vi "Calculate New Account Balance.vi"(6 "Amount":string, 8 "error in (no error)":errorcluster, 11 "Bank Account in":refnum<class "Bank Account.lvclass">) -> (0 "error out":errorcluster, 3 "Bank Account out":refnum<class "Bank Account.lvclass">, 4 "Sufficient Funds?":bool)   [LabVIEW 2016, in "CLD Exam - ATM.lvlib" / "Bank Account.lvclass"]
uses:
  Bank Account.lvclass
  Bank Account.lvclass/Bank Account.ctl
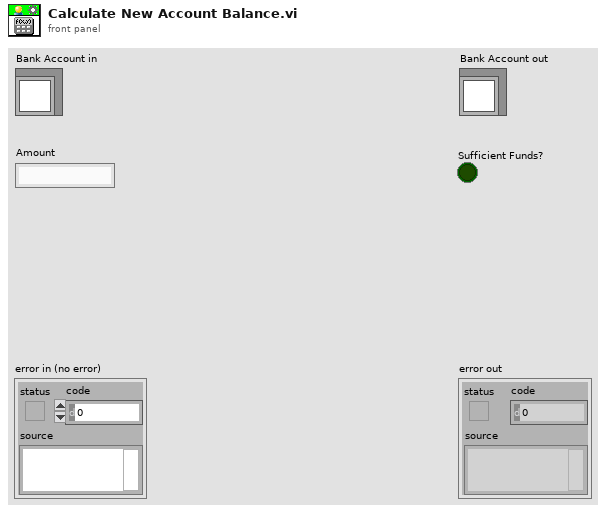
[diagram p1: front panel]
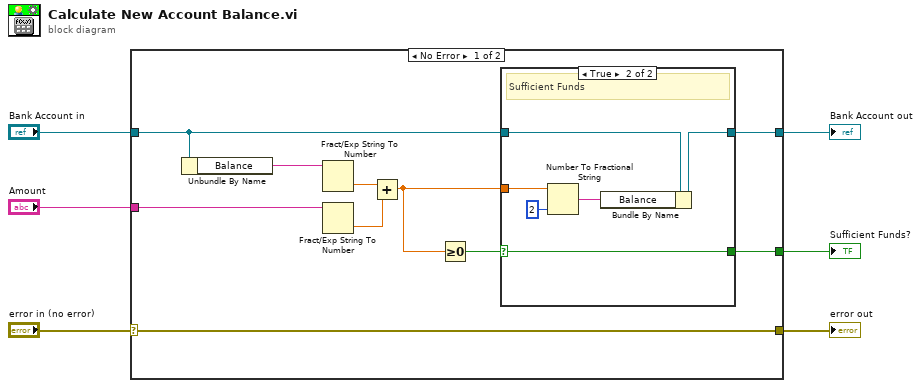
[diagram p0: block diagram]
diagram:
  n1 = case shown="No Error" "error in (no error)" {
    selector: "error in (no error)" -> [w16 w26]
    tunnel: [w16 w26] -> w5
    tunnel: [w8 w25] -> w3
    tunnel: "Bank Account in" -> [w9 w25]
    tunnel: "Amount" -> [w12 _]
    tunnel: [w7 _] -> w1
    frame No Error {
      n2 = Unbundle By Name(w9) -> ("Balance"=w13:string)
      n3 = Fract/Exp String To Number(string=w13) -> (number=w15:dbl)  [unwired: 3 in, 1 out]
      n4 = Fract/Exp String To Number(string=w12) -> (number=w14:dbl)  [unwired: 3 in, 1 out]
      n5 = Add(x=w15, y=w14) -> (x+y=w10:dbl)
      n6 = Greater Or Equal To 0?(x=w10) -> (x >= 0?=w11:bool)
      n7 = case shown="True" w11 {
        selector: w11 -> [w17 w19]
        tunnel: w10 -> [_ w23]
        tunnel: [w18 w21] -> w8
        tunnel: w9 -> [w18 w22]
        tunnel: [w17 w19] -> w7
        frame False {
          # "Insufficient Funds"
        }
        frame True {
          # "Sufficient Funds"
          n8 = Number To Fractional String(number=w23, precision (6)=i16 2) -> (F-format string=w20:string)  [unwired: 2 in]
          n9 = Bundle By Name(cluster=w22, "Balance"=w20) -> (w21:refnum<class "Bank Account.lvclass">)
        }
      }
    }
    frame Error {
    }
  }
  "error out" <- w5
  "Bank Account out" <- w3
  "Sufficient Funds?" <- w1
